vi "GetPinNumbering.vi"(6 "error in":errorcluster) -> (0 "error out":errorcluster, 4 "Pin Numbering":T1)   [LabVIEW 2014, in "Raspberry Pi Compatible Compiler for LabVIEW.lvlib" / "GPIO.lvlib"]
doc: "This VI returns the IO pin numbering system currently being used. BCM numbers refer to channel numbers on the Broadcom SOC. Board numbers refer to the pin numbers of the P1 header."
uses:
  GPIO.lvlib
  controls/PinNumbering.ctl
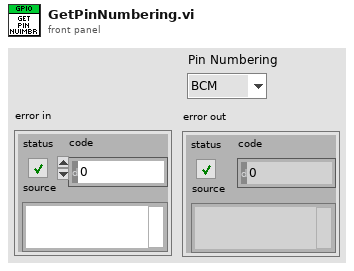
[diagram p1: front panel]
types:
  T1 = typedef "Raspberry Pi Compatible Compiler for LabVIEW.lvlib/GPIO.lvlib/PinNumbering.ctl" = enum16{"BCM", "Board"}
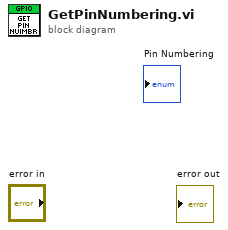
[diagram p0: block diagram]
diagram:
